vi "Histogram.vi"(11 "8-bit pixmap":u8[][](array[numeric])) -> (3 "Histogram Graph":T1(graph) caption="直方图")   [LabVIEW 2011]
uses:
  <vilib>/Analysis/NI_AALBase.lvlib
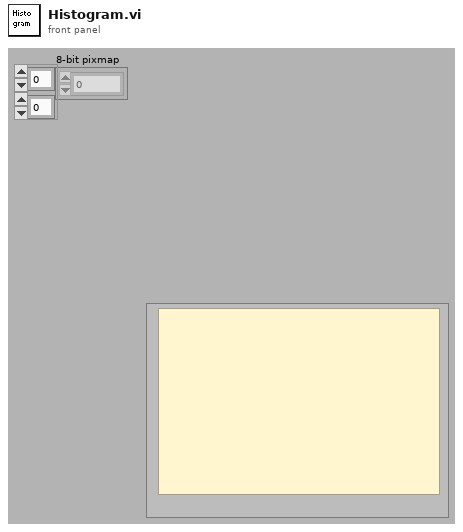
[diagram p1: front panel]
types:
  T1 = cluster{"X Values":dbl[], "Histogram: h(x)":i32[]}
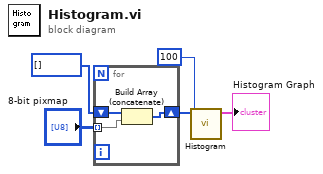
[diagram p0: block diagram]
diagram:
  n1 = for {
    shift-right: [w7] -> w3
    shift-left: u8[] [] ("Image Pixels (U8)") -> [w8]
    tunnel: "8-bit pixmap" -> [w6] mode=indexing
    n2 = Build Array (concatenate)(w8, w6) -> (w7:u8[])
  }
  n3 = call <vilib>:"Histogram.vi"("intervals"=100, "X"=w3) -> ("Histogram Graph"=→"Histogram Graph":T1)  [unwired: 9 out]
